vi "test Separate Inline and Async.vi"(8 "error in (no error)":errorcluster, 11 "TestCase in":refnum<class "Configuration Tests.lvclass">) -> (0 "error out":errorcluster, 3 "TestCase out":refnum<class "Configuration Tests.lvclass">)   [LabVIEW 2017, in "Configuration Tests.lvclass"]
uses:
  Configuration Tests.lvclass
  Mock Classes/Transfer Group/Mock Transfer Group.lvclass
  C:/Git/DSF/Data Sharing Framework Core/Classes/Transfer Group/Transfer Group.lvclass
  <vilib>/addons/_JKI Toolkits/VI Tester/TestCase.llb/TestCase.lvclass
  Classes/Transfer Group/Transfer Group.lvclass
  C:/Program Files (x86)/National Instruments/LabVIEW 2017/vi.lib/addons/_JKI Toolkits/VI Tester/TestCase.llb/TestCase.lvclass
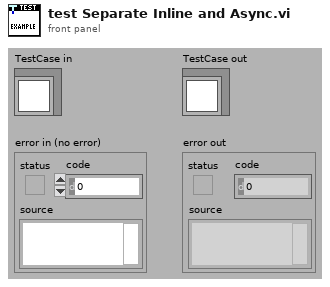
[diagram p1: front panel]
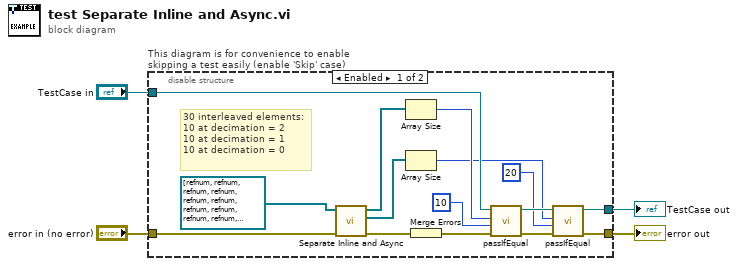
[diagram p0: block diagram]
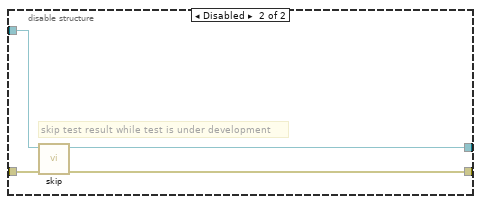
[diagram p2: hidden frame]
diagram:
  n1 = disable-structure "This diagram is for convenience to enable skipping a test easily (enable 'Skip' case)" shown="Enabled" {
    disable-tunnel: "TestCase in" -> [w12 w23]
    disable-tunnel: [w9 w21] -> w1
    disable-tunnel: [w11 w22] -> w3
    disable-tunnel: "error in (no error)" -> [w19 w20]
    frame Enabled {
      # "30 interleaved elements:\n10 at decimation = 2\n10 at decimation = 1\n10 at decimation = 0"
      n2 = call "Separate Inline and Async.vi"("error in (no error)"=w19, "Transfer Groups"=refnum<class "Mock Transfer Group.lvclass">[] [refnum, refnum, refnum, refnum, refnum, refnum, refnum, refnum, refnum, refnum, refnum, refnum, refnum, refnum, refnum, refnum, refnum, refnum, refnum, refnum, refnum, refnum, refnum, refnum, refnum, refnum, refnum, refnum, refnum, refnum] ("interleaved array")) -> ("error out"=w18:errorcluster, "Async Transfer Groups"=w14:refnum<class "Transfer Group.lvclass">[], "Inline Transfer Groups"=w15:refnum<class "Transfer Group.lvclass">[])  [unwired: 7 in]
      n3 = Array Size(array=w15) -> (size(s)=w8:i32)
      n4 = Array Size(array=w14) -> (size(s)=w6:i32)
      n5 = Merge Errors(w18) -> (w17:errorcluster)
      n6 = call-dynamic "passIfEqual.vi"("error in (no error)"=w17, "y"=10 ("size(s)"), "x"=w8, "TestCase in"=w12) -> ("error out"=w13:errorcluster, "TestCase out"=w10:refnum<class "Configuration Tests.lvclass">)  [unwired: 6 in]
      n7 = call-dynamic "passIfEqual.vi"("error in (no error)"=w13, "y"=20 ("size(s)"), "x"=w6, "TestCase in"=w10) -> ("error out"=w11:errorcluster, "TestCase out"=w9:refnum<class "Configuration Tests.lvclass">)  [unwired: 6 in]
    }
    frame Disabled {
      # "skip test result while test is under development"
      n8 = call <vilib>:"skip.vi"("error in (no error)"=w20, "TestCase in"=w23) -> ("error out"=w22:errorcluster, "TestCase out"=w21:refnum<class "Configuration Tests.lvclass">)  [unwired: 8 in]
    }
  }
  "error out" <- w3
  "TestCase out" <- w1
